vi "ml_Initialize Centroids.vi"(8 "error in (no error)":errorcluster, 9 "# of classes":i32=1, 10 "Centroids in":dbl[][](array[numeric]), 11 "Samples":dbl[][](array[numeric])) -> (0 "error out":errorcluster, 2 "Centroids out":dbl[][](array[numeric]), 3 "Samples dup":dbl[][](array[numeric]))   [LabVIEW 2013, in "NILabs_MLT.lvlib"]
uses:
  <vilib>/addons/Machine Learning/NILabs_MLT.lvlib
  <vilib>/Analysis/1siggen.llb/Riffle Array (I32) (obs 2012).vi
  <vilib>/Analysis/NI_AALBase.lvlib
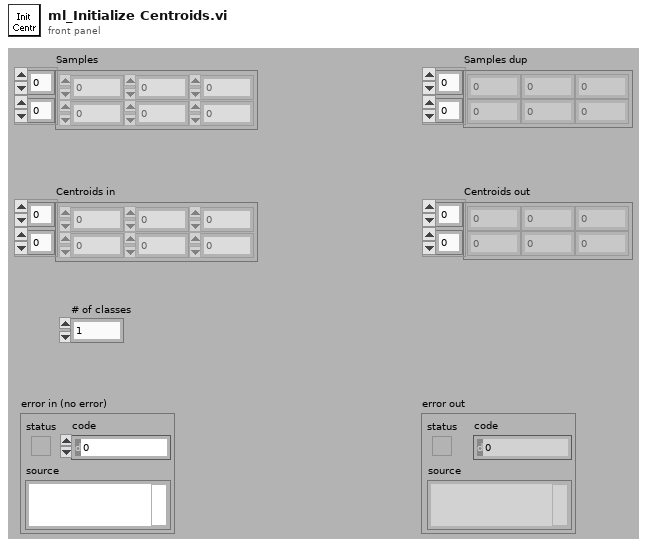
[diagram p1: front panel]
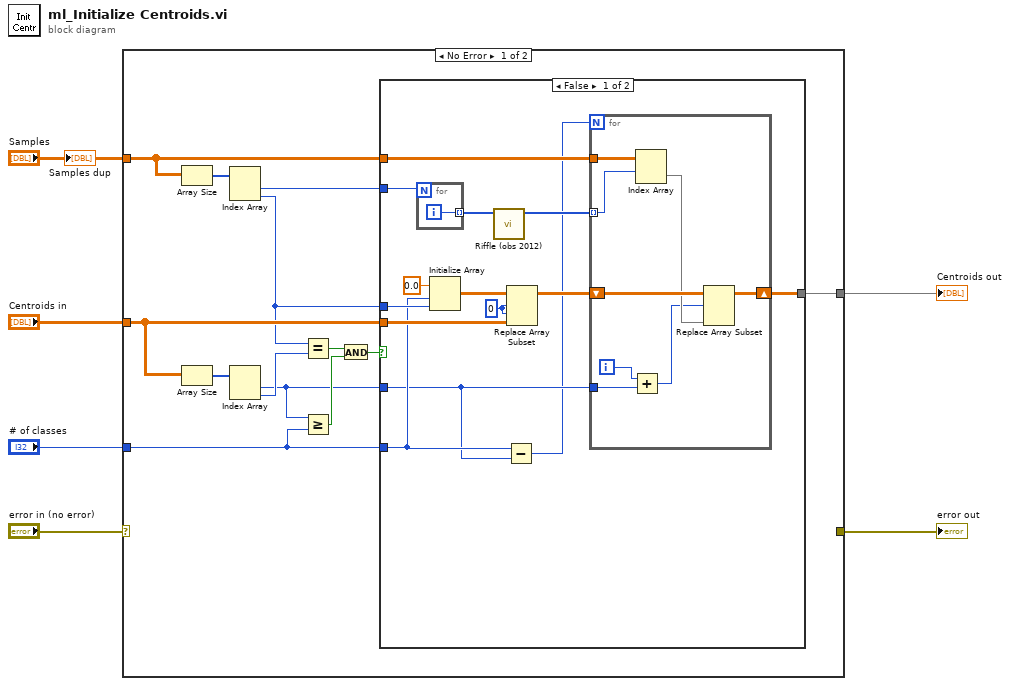
[diagram p0: block diagram]
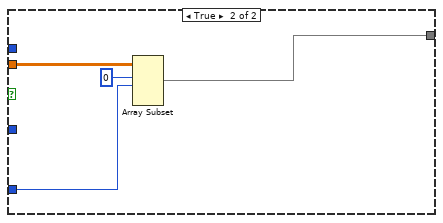
[diagram p2: hidden frame]
diagram:
  n1 = case shown="No Error" "error in (no error)" {
    selector: "error in (no error)" -> [_ w47]
    tunnel: "Samples" -> [w13 _]
    tunnel: "Centroids in" -> [w12 _]
    tunnel: "# of classes" -> [w10 _]
    tunnel: [w7 _] -> w2
    tunnel: [_ w47] -> w1
    frame No Error {
      n2 = Array Size(array=w13) -> (size(s)=w19:i32[])
      n3 = Array Size(array=w12) -> (size(s)=w18:i32[])
      n4 = Index Array(array=w19) -> (element #1=w9:i32, element #2=w8:i32)  [unwired: 2 in]
      n5 = Index Array(array=w18) -> (element #1=w11:i32, element #2=w17:i32)  [unwired: 2 in]
      n6 = Equal?(x=w8, y=w17) -> (x = y?=w16:bool)
      n7 = Greater Or Equal?(x=w11, y=w10) -> (x >= y?=w15:bool)
      n8 = And(x=w16, y=w15) -> (x .and. y?=w14:bool)
      n9 = case shown="False" w14 {
        tunnel: w13 -> [w31 _]
        tunnel: w12 -> [w26 w46]
        tunnel: w11 -> [w21 _]
        tunnel: w10 -> [w22 w44]
        tunnel: [w23 w43] -> w7
        tunnel: w9 -> [w33 _]
        tunnel: w8 -> [w29 _]
        frame False {
          w25 = 0 ("index (row)")
          n10 = for {
            N: w33 -> [_]
            tunnel: [w42] -> w32 mode=indexing
            i -> [w42]
          }
          n11 = Initialize Array(0.0 ("element"), w22, w29) -> (w27:dbl[][])
          n12 = call-poly <vilib>:"Riffle (obs 2012).vi"("X"=w32) -> ("Riffled {X}"=w30:i32[])  [unwired: 8 in, 2 out]
          n13 = Subtract(x=w22, y=w21) -> (x-y=w20:i32)
          n14 = Replace Array Subset(array=w27, new element=w26, index (row)=w25, index (col)=w25) -> (w24:dbl[][])
          n15 = for {
            N: w20 -> [_]
            shift-right: [w39] -> w23
            shift-left: w24 -> [w40]
            tunnel: w31 -> [w41]
            tunnel: w30 -> [w34] mode=indexing
            tunnel: w21 -> [w37]
            i -> [w36]
            n16 = Add(x=w36, y=w37) -> (x+y=w35:i32)
            n17 = Index Array(array=w41, index (row)=w34) -> (element=w38:dbl[])  [unwired: 1 in]
            n18 = Replace Array Subset(array=w40, new element=w38, index (row)=w35) -> (w39:dbl[][])  [unwired: 1 in]
          }
        }
        frame True {
          n19 = Array Subset(array=w46, index (row)=0 ("index"), length (row)=w44) -> (w43:dbl[][])  [unwired: 2 in]
        }
      }
    }
    frame Error {
    }
  }
  "error out" <- w1
  "Centroids out" <- w2
  "Samples dup" <- "Samples"
